vi "Dart.vi"(9 "Button 1":bool, 11 "Axis 1":dbl) -> ()   [LabVIEW 2015]
uses:
  Robot Global Data.vi
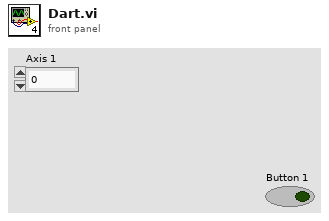
[diagram p1: front panel]
types:
  T1 = typedef "WPI_MotorControlDeviceRef.ctl" = cluster{"DeviceStatus":errorcluster, "Type":T2, "PWM":cluster{"PWM Channel":T3, "DeadBand":T4}, "CAN":cluster{"Device Number":u8, "Control Mode":T5, "Semaphore":T6, "Max Vout":dbl, "TalonSRX Control Mode":T7}, "Invert":bool}
  T2 = typedef "WPI_MotorControlType.ctl" = enum16{"PWM", "CAN", "CANTalonSRX"}
  T3 = typedef "FPGA_DIOPWMChannel.ctl" = enum8{"PWM 0", "PWM 1", "PWM 2", "PWM 3", "PWM 4", "PWM 5", "PWM 6", "PWM 7", "PWM 8", "PWM 9", "PWM MXP 0", "PWM MXP 1", "PWM MXP 2", "PWM MXP 3", "PWM MXP 4", "PWM MXP 5", "PWM MXP 6", "PWM MXP 7", "PWM MXP 8", "PWM MXP 9", "Invalid"}
  T4 = typedef "WPI_PWMDeadband.ctl" = cluster{"Name":string, "maxPositivePwm":i32, "minPositivePwm":i32, "centerPwm":i32, "maxNegativePwm":i32, "minNegativePwm":i32, "angularRange":u16}
  T5 = typedef "WPI_CANJaguar_ControlMode.ctl" = enum8{"Percent VBus", "Current", "Speed", "Position", "Voltage"}
  T6 = typedef "Semaphore RefNum" = refnum<k1>
  T7 = typedef "WPI_CANTalonSRX_APIControlMode.ctl" = enum8{"Percent VBus", "Speed", "Position", "Slave", "Unchanged / Invalid", "Voltage Compensation", "Current", "Motion Profile"}
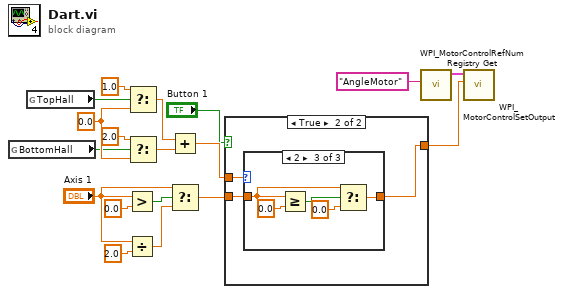
[diagram p0: block diagram]
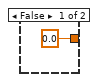
[diagram p2: hidden frame]
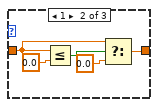
[diagram p4: hidden frame]
diagram:
  w15 = 0.0 ("f")
  n1 = global read "Robot Global Data.vi" "BottomHall"() -> (w1:bool)
  n2 = global read "Robot Global Data.vi" "TopHall"() -> (w2:bool)
  n3 = Greater?(x="Axis 1", y=0.0) -> (0:w12:bool)
  n4 = Divide(x="Axis 1", y=2.0) -> (x/y=w9:dbl)
  n5 = Select(t=1.0, s=w2, f=w15) -> (s? t:f=w14:dbl)
  n6 = Select(t=2.0, s=w1, f=w15) -> (s? t:f=w13:dbl)
  n7 = Add(x=w14, y=w13) -> (x+y=w8:dbl)
  n8 = Select(t="Axis 1", s=w12, f=w9) -> (s? t:f=w7:dbl)
  n9 = case shown="True" "Button 1" {
    tunnel: w8 -> [_ w22]
    tunnel: w7 -> [_ w21]
    tunnel: [0.0 ("f") w20] -> w6
    frame False {
    }
    frame True {
      n10 = case shown="2" w22 {
        tunnel: w21 -> [w23 w25 w29]
        tunnel: [w23 w24 w30] -> w20
        frame 0, Default {
        }
        frame 1 {
          n11 = Less Or Equal?(x=w25, y=0.0) -> (x <= y?=w26:bool)
          n12 = Select(t=w25, s=w26, f=0.0) -> (s? t:f=w24:dbl)
        }
        frame 2 {
          n13 = Greater Or Equal?(x=w29, y=0.0) -> (x >= y?=w31:bool)
          n14 = Select(t=w29, s=w31, f=0.0) -> (s? t:f=w30:dbl)
        }
      }
    }
  }
  n15 = call <vilib>:"WPI_MotorControlRefNum Registry Get.vi"("refnum name"="AngleMotor") -> ("MotorControlDevRef"=w5:T1)  [unwired: 9 in, 1 out]
  n16 = call <vilib>:"WPI_MotorControlSetOutput.vi"("Output"=w6, "MotorControlDevRef"=w5) -> ()  [unwired: 7 in, 3 out]
